vi "FTW-ProjectItemManager-Get.vi"(0 "Project Item Manager":refnum<class "FTW-ProjectItemManager.lvclass">, 5 "Tag":string, 7 "Default Value":string="NULL", 11 "error in":errorcluster) -> (4 "Project Item Manager out":refnum<class "FTW-ProjectItemManager.lvclass">, 8 "Value":string, 15 "error out":errorcluster)   [LabVIEW 2013, in "FTW-ProjectItemManager.lvclass"]
uses:
  FTW-ProjectItemManager.lvclass
  FTW-ProjectItemManager.lvclass/FTW-ProjectItemManager.ctl
  Core/Collection/FTW-Collection.lvclass
panel:
  # "Inputs"
  # "Outputs"
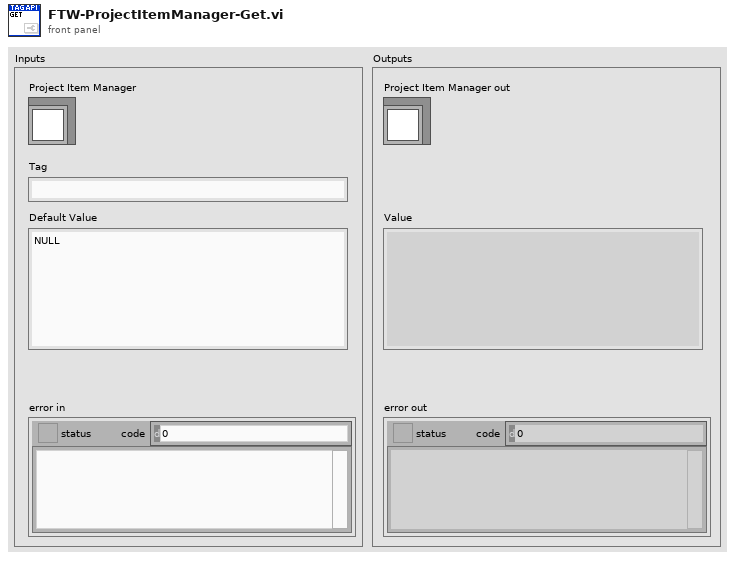
[diagram p1: front panel]
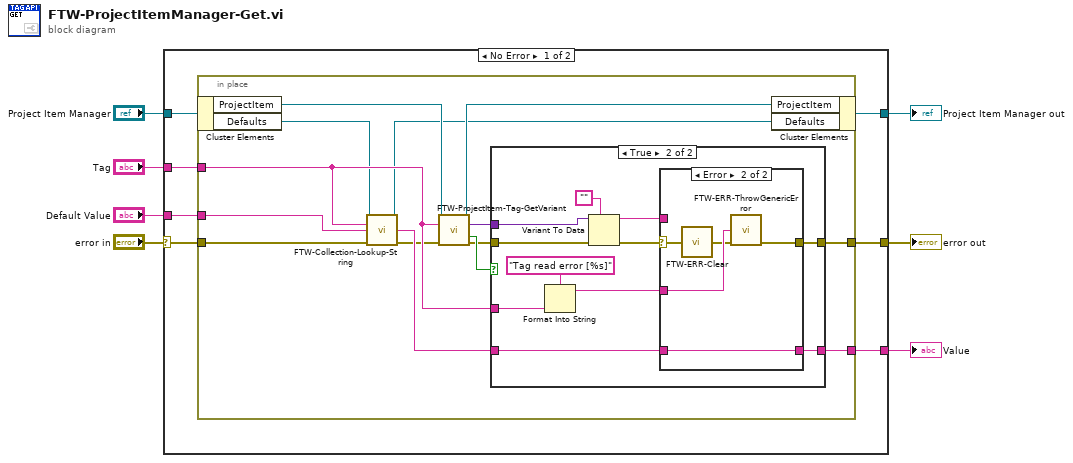
[diagram p0: block diagram]
diagram:
  n1 = case shown="No Error" "error in" {
    selector: "error in" -> [w13 w50]
    tunnel: [w10 w50] -> w7
    tunnel: "Tag" -> [w11 _]
    tunnel: [w14 _] -> w4
    tunnel: "Default Value" -> [w12 _]
    tunnel: "Project Item Manager" -> [w9 w49]
    tunnel: [w8 w49] -> w1
    frame No Error {
      n2 = in-place {
        in-place-border: [w28] -> w14
        in-place-border: w13 -> [w20]
        in-place-border: w12 -> [w22]
        in-place-border: w11 -> [w23]
        in-place-border: [w15] -> w10
        n3 = in-place-cluster #1(w9) -> ("ProjectItem"=w25:refnum<vi>, "Defaults"=w18:refnum<class "FTW-Collection.lvclass">)
        n4 = call "FTW-Collection-Lookup-String.vi"("Collection"=w18, "Key"=w23, "Default Value"=w22, "error in"=w20) -> ("Collection out"=w17:refnum<class "FTW-Collection.lvclass">, "Value"=w21:string, "error out"=w19:errorcluster)  [unwired: 8 in, 1 out]
        n5 = call "FTW-ProjectItem-Tag-GetVariant.vi"("ProjectItem"=w25, "Tag Name"=w23, "error in"=w19) -> ("ProjectItem out"=w24:refnum<vi>, "Tag Value"=w26:variant, "Exists?"=w27:bool, "error out"=w16:errorcluster)  [unwired: 8 in, 1 out]
        n6 = case shown="True" w27 {
          tunnel: [w30 w41] -> w28
          tunnel: w26 -> [_ w40]
          tunnel: w16 -> [w29 w38]
          tunnel: w23 -> [_ w36]
          tunnel: w21 -> [w30 w35]
          tunnel: [w29 w31] -> w15
          frame False {
          }
          frame True {
            n7 = Format Into String(format string="Tag read error [%s]", w36) -> (resulting string=w32:string)  [unwired: 2 in, 1 out]
            n8 = Variant To Data(error in=w38, type="", Variant=w40) -> (data=w39:string, error out=w33:errorcluster)
            n9 = case shown="Error" w33 {
              selector: w33 -> [w42 w46]
              tunnel: [w43 w48] -> w41
              tunnel: w39 -> [w43 _]
              tunnel: w35 -> [_ w48]
              tunnel: w32 -> [_ w47]
              tunnel: [w42 w44] -> w31
              frame No Error {
              }
              frame Error {
                n10 = call "FTW-ERR-Clear.vi"("error to snuff"=w46) -> ("no error"=w45:errorcluster)
                n11 = call "FTW-ERR-ThrowGenericError.vi"("Error Message"=w47, "error in"=w45) -> ("error out"=w44:errorcluster)  [unwired: 13 in]
              }
            }
          }
        }
        n12 = in-place-cluster #1("ProjectItem"=w24, "Defaults"=w17) -> (w8:refnum<class "FTW-ProjectItemManager.lvclass">)
      }
    }
    frame Error {
    }
  }
  "error out" <- w7
  "Value" <- w4
  "Project Item Manager out" <- w1
